vi "Init Data.vi"(10 "Data":T1) -> (3 "Msg out":refnum<class "Msg.lvclass">)   [LabVIEW 2020, in "TcpServerHello.lvlib" / "Msg.lvclass"]
uses:
  Msg.lvclass
  Data.ctl
  ConnectStatus/Enumeration.ctl
  Msg.lvclass/Msg.ctl
  TcpServerHello.lvlib
  ConnectStatus/ConnectStatus.lvlib
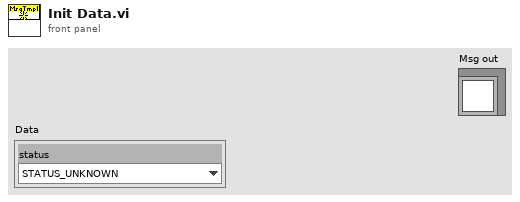
[diagram p1: front panel]
types:
  T1 = typedef "TcpServerHello.lvlib/Data.ctl" = cluster{"status":T2}
  T2 = typedef "ConnectStatus.lvlib/Enumeration.ctl" = enum16{"STATUS_UNKNOWN", "STATUS_SUCCESS", "STATUS_ERROR", "STATUS_BAD_CONFIG", "STATUS_BAD_SYSTEM", "STATUS_BAD_CLUSTER", "STATUS_NOT_ALLOWED"}
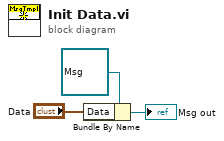
[diagram p0: block diagram]
diagram:
  n1 = Bundle By Name(cluster=refnum<class "Msg.lvclass"> refnum ("Msg out"), "Data"="Data") -> (→"Msg out":refnum<class "Msg.lvclass">)
